vi "DAC Configure.vi"(8 "error in":errorcluster, 11 "DAC HS Vib in":refnum<class "DAC HS Vib.lvclass">) -> (0 "error out":errorcluster, 3 "DAC HS Vib out":refnum<class "DAC HS Vib.lvclass">)   [LabVIEW 2019, in "DAC.lvlib" / "DAC HS Vib.lvclass"]
uses:
  DAC HS Vib.lvclass
  C:/Users/krio/Documents/LV_Projects/test-stand/App/DAC/DAC.lvclass
  DAC.lvclass/DAC.ctl
  DAC HS Vib.lvclass/DAC HS Vib.ctl
  <vilib>/DAQmx/create/scale.llb/DAQmx Create Scale (Map Ranges).vi
  <vilib>/DAQmx/create/channels.llb/DAQmx Create Channel (AI-Voltage-Basic).vi
  <vilib>/DAQmx/configure/timing.llb/DAQmx Timing (Sample Clock).vi
  DAC.lvclass
  <vilib>/DAQmx/create/channels.llb/DAQmx Create Channel (AI-Current-Basic).vi
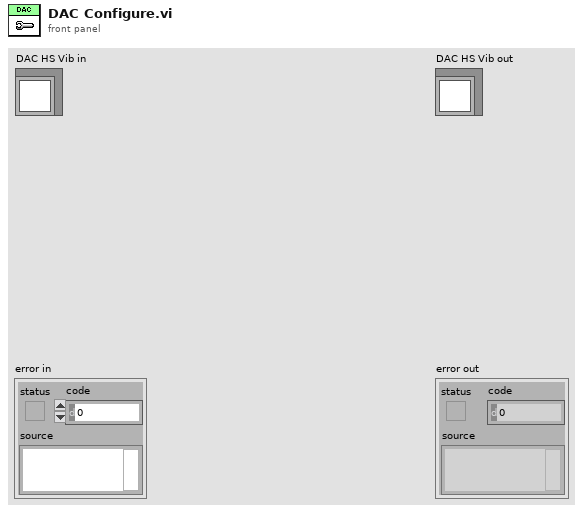
[diagram p1: front panel]
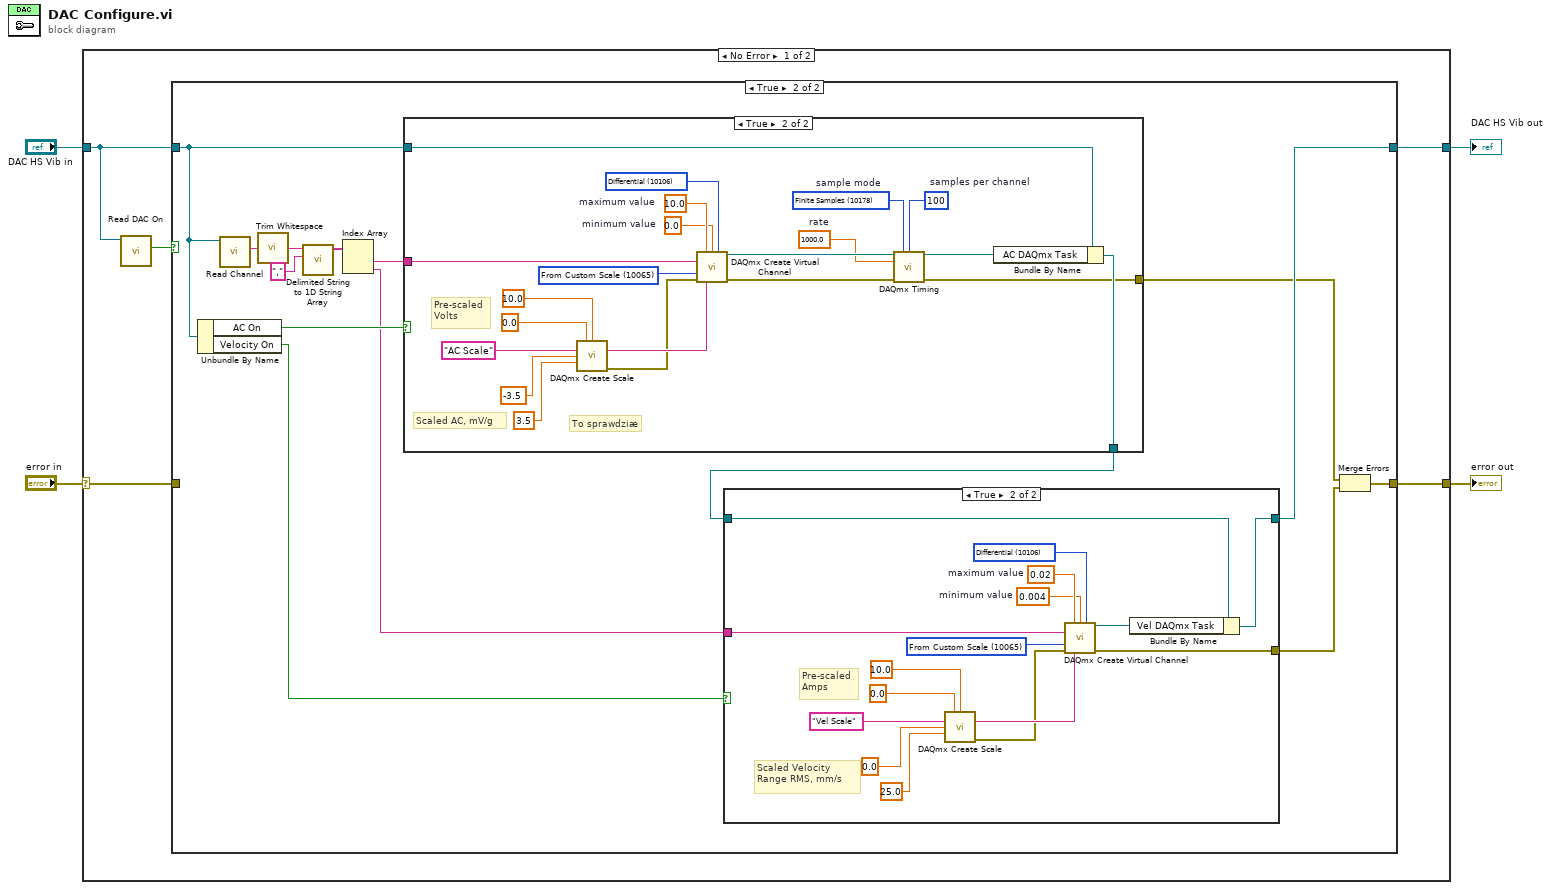
[diagram p0: block diagram]
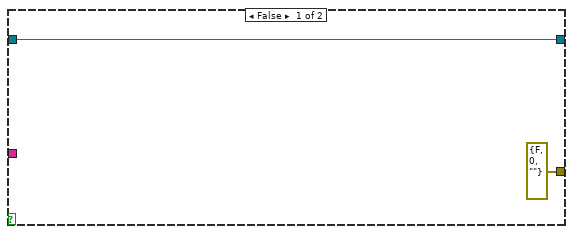
[diagram p3: hidden frame]
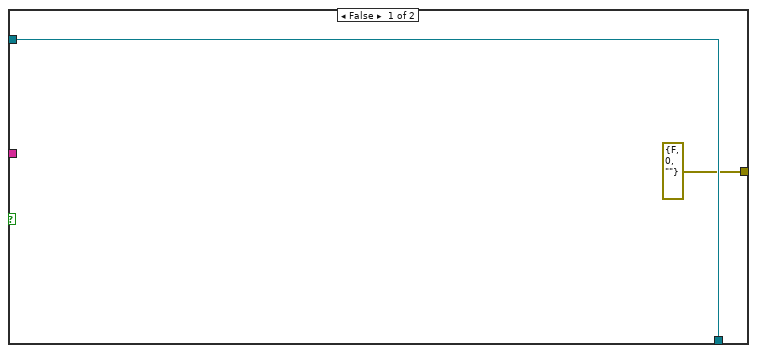
[diagram p4: hidden frame]
diagram:
  n1 = case shown="No Error" "error in" {
    selector: "error in" -> [w6 w68]
    tunnel: [w5 w68] -> w4
    tunnel: [w7 w67] -> w3
    tunnel: "DAC HS Vib in" -> [w9 w67]
    frame No Error {
      n2 = call "Read DAC On.vi"("DAC in"=w9) -> ("DAC On"=w8:bool)  [unwired: 8 in, 2 out]
      n3 = case shown="True" w8 {
        tunnel: w9 -> [w11 w22]
        tunnel: [w11 w16] -> w7
        tunnel: w6 -> [w10 _]
        tunnel: [w10 w14] -> w5
        frame False {
        }
        frame True {
          n4 = Unbundle By Name(w22) -> ("AC On"=w25:bool, "Velocity On"=w19:bool)
          n5 = call "Read Channel.vi"("DAC in"=w22) -> ("Channel"=w24:string)  [unwired: 8 in, 2 out]
          n6 = call <vilib>:"Trim Whitespace.vi"("string"=w24) -> ("trimmed string"=w21:string)  [unwired: 1 in]
          n7 = call <vilib>:"Delimited String to 1D String Array.vi"("delimiter"=",", "delimited string"=w21) -> ("string array"=w20:string[])  [unwired: 9 in]
          n8 = Index Array(array=w20) -> (element #1=w17:string, element #2=w15:string)  [unwired: 2 in]
          n9 = case shown="True" w25 {
            tunnel: w22 -> [w45 w66]
            tunnel: [w45 w48] -> w18
            tunnel: w17 -> [_ w47]
            tunnel: [errorcluster {"status"=FALSE, "code"=0, "source"=""} ("error out") w46] -> w13
            frame False {
            }
            frame True {
              w57 = 10106 items=["Default"=-1, "RSE"=10083, "NRSE"=10078, "Differential"=10106, "Pseudodifferential"=12529] ("input terminal configuration")
              w58 = 0.0  # minimum value
              w59 = 10.0  # maximum value
              w60 = 100  # samples per channel
              w61 = 1000.0  # rate
              w62 = 10178 items=["Finite Samples"=10178, "Continuous Samples"=10123, "Hardware Timed Single Point"=12522]  # sample mode
              w65 = 10065 items=["Volts"=10348, "From Custom Scale"=10065] ("units")
              # "To sprawdziæ"
              # "Scaled AC, mV/g"
              # "Pre-scaled\nVolts"
              n10 = call-poly <vilib>:"DAQmx Create Scale.vi"("pre-scaled minimum"=0.0, "pre-scaled maximum"=10.0, "name"="AC Scale", "scaled minimum"=-3.5, "scaled maximum"=3.5) -> ("scale out"=w51:tag, "error out"=w50:errorcluster)  [unwired: 9 in]
              n11 = call-poly <vilib>:"DAQmx Create Virtual Channel.vi"("maximum value"=w59, "minimum value"=w58, "input terminal configuration"=w57, "physical channels"=w47, "units"=w65, "error in"=w50, "custom scale name"=w51) -> ("task out"=w64:refnum<k21>, "error out"=w63:errorcluster)  [unwired: 7 in]
              n12 = call-poly <vilib>:"DAQmx Timing.vi"("task/channels in"=w64, "sample mode"=w62, "samples per channel"=w60, "rate"=w61, "error in"=w63) -> ("task out"=w49:refnum<k21>, "error out"=w46:errorcluster)  [unwired: 9 in]
              n13 = Bundle By Name(cluster=w66, "AC DAQmx Task"=w49) -> (w48:refnum<class "DAC HS Vib.lvclass">)
            }
          }
          n14 = case shown="True" w19 {
            tunnel: [w27 w43] -> w16
            tunnel: w18 -> [w27 w42]
            tunnel: w15 -> [_ w29]
            tunnel: [errorcluster {"status"=FALSE, "code"=0, "source"=""} ("error out") w28] -> w12
            frame False {
            }
            frame True {
              w37 = 10106 items=["Default"=-1, "RSE"=10083, "NRSE"=10078, "Differential"=10106, "Pseudodifferential"=12529] ("input terminal configuration")
              w38 = 0.004  # minimum value
              w39 = 0.02  # maximum value
              w41 = 10065 items=["Volts"=10348, "From Custom Scale"=10065] ("units")
              # "Scaled Velocity Range RMS, mm/s"
              # "Pre-scaled\nAmps"
              n15 = call-poly <vilib>:"DAQmx Create Scale.vi"("pre-scaled minimum"=0.0, "pre-scaled maximum"=10.0, "name"="Vel Scale", "scaled minimum"=0.0, "scaled maximum"=25.0) -> ("scale out"=w31:tag, "error out"=w30:errorcluster)  [unwired: 9 in]
              n16 = call-poly <vilib>:"DAQmx Create Virtual Channel.vi"("maximum value"=w39, "minimum value"=w38, "input terminal configuration"=w37, "physical channels"=w29, "units"=w41, "error in"=w30, "custom scale name"=w31) -> ("task out"=w40:refnum<k21>, "error out"=w28:errorcluster)  [unwired: 7 in]
              n17 = Bundle By Name(cluster=w42, "Vel DAQmx Task"=w40) -> (w43:refnum<class "DAC HS Vib.lvclass">)
            }
          }
          n18 = Merge Errors(w13, w12) -> (w14:errorcluster)
        }
      }
    }
    frame Error {
    }
  }
  "error out" <- w4
  "DAC HS Vib out" <- w3
